vi "Main_Transmitter.vi"(8 "error in (no error)":errorcluster, 10 "Packet Parameters in":T3={"Length of sync sequence (50)"=50, "Number of message bits"=2048, "Number of guardbits"=30, "Sync PN sequence order (31)"=31, "Number of header bits"=16, "Packet Pad [samples]"=200}, 11 "QPSK System Parameters":T4={"Samples per Symbol"=8, "symbol map"=[], "Differential PSK"=enum."enable", "PSK type"=0, "M-PSK"=8} {"PSK type" items=["normal", "shifted", "offset"]; "symbol map" format="%.3f"}) -> (0 "error out":errorcluster)   [LabVIEW 2014]
uses:
  <vilib>/addons/Modulation/Digital/General/MT Generate Bits (Galois, PN Order).vi
  <vilib>/addons/Modulation/Digital/Support/Common/Validators/mod_Generate Bits Validate.vi
  <vilib>/addons/Modulation/Analog/support/mod_Set Error Source.vi
  <vilib>/addons/Modulation/Digital/General/subVIs/mod_Generate Bits PN Sequence.vi
  <vilib>/addons/Modulation/Digital/General/MT Format Eye Diagram (complex).vi
  <instrlib>/niUSRP/niUSRP Write Tx Data (CDB Cluster).vi
  <vilib>/addons/Modulation/niDMT.lvlib
panel:
  out "Time to modulate packet [ms]":dbl
  in  "Test Setup":T1={"Packets to send"=100, "Queue Length"=10, "PN sequence order (9)"=9}
  in  "I/Q (I)":enum16{"I", "Q"}(ring) caption="Eye Diagram I/Q"
  out "Eye Diagram":cluster{"t0":dbl, "dt":dbl, "Y":dbl[]}[](graph)
  in  "autoscale":bool
  out "Constellation Graph":T2(graph)
  out "Frame transfer time [ms]":dbl
  out "Frame length [samples]":i32
  out "Effective bit rate [bits/s]":dbl
  out "Real Frames Sent":i32
  out "Blank Frames Sent":i32
  out "Time to transfer packet [ms]":dbl
  in  "stop 2":bool caption="stop"
  in  "Bits per sample":i32=16
  in  "Audio record time/delay (ms)":i32=200
  in  "Audio sample rate (Fs)":i32=6000
  in  "filter parameters":T5={"Alpha"=0.5, "Filter Length"=6, "TX Filter"=enum."Root Raised Cos"} {"Alpha" format="%.2f"}
  in  "USRP IP address":refnum<k15>="192.168.10.1"
  in  "Tx Parameters":T6={"Tx IQ Sampling\nRate [s/sec]"=400000.0, "Tx Frequency [Hz]"=2450000000.0, "Tx Gain [dB]"=0.0, "Tx Antenna"="TX1"} {"Tx Gain [dB]" format="%#.6p"; "Tx Frequency [Hz]" format="%#.6p"; "Tx IQ Sampling\nRate [s/sec]" format="%#.6p"}
  out "Actual Tx Parameters":T6={"Tx IQ Sampling\nRate [s/sec]"=400000.0, "Tx Frequency [Hz]"=915000000.0, "Tx Gain [dB]"=0.0, "Tx Antenna"="TX1"} {"Tx Gain [dB]" format="%#.6p"; "Tx Frequency [Hz]" format="%#.6p"; "Tx IQ Sampling\nRate [s/sec]" format="%#.6p"}
  # "Calculated values"
  # "Measurements"
  # "Graph Setup"
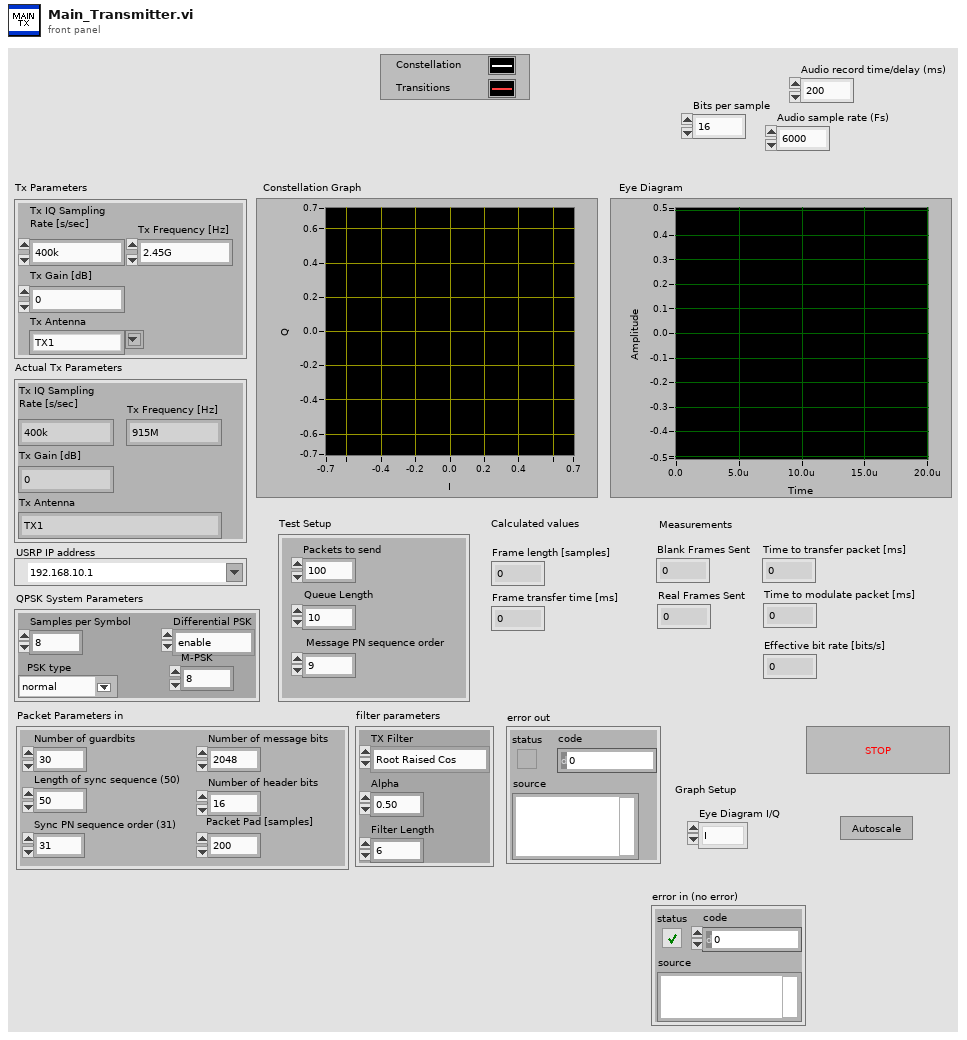
[diagram p1: front panel]
types:
  T1 = cluster{"Packets to send":i32, "Queue Length":i32, "PN sequence order (9)":i32}
  T2 = cluster{"Decimated Array":dbl[], "Decimated Array":dbl[]}[]
  T3 = cluster{"Length of sync sequence (50)":i32, "Number of message bits":i32, "Number of guardbits":i32, "Sync PN sequence order (31)":i32, "Number of header bits":i32, "Packet Pad [samples]":i32}
  T4 = cluster{"Samples per Symbol":i32, "symbol map":cdb[], "Differential PSK":enum16{"disable", "enable"}, "PSK type":u16, "M-PSK":i32}
  T5 = cluster{"Alpha":dbl, "Filter Length":i32, "TX Filter":enum16{"none", "Raised Cosine", "Root Raised Cos", "Gaussian"}}
  T6 = cluster{"Tx IQ Sampling\nRate [s/sec]":dbl, "Tx Frequency [Hz]":dbl, "Tx Gain [dB]":dbl, "Tx Antenna":string}
  T7 = cluster{"samples per symbol (16)":i32, "symbol map":cdb[], "differential PSK":enum16{"disable", "enable"}, "PSK type":u16}
  T8 = cluster{"s? t:f":cluster{"t0":dbl, "dt":dbl, "Y":cdb[]}, i32}
  T9 = typedef "niAMT.lvlib/Complex Data Waveform.ctl" = cluster{"t0":dbl, "dt":dbl, "Y":cdb[]}
  T10 = cluster{"constellation":dbl[], "oversampled data":dbl[]}[]
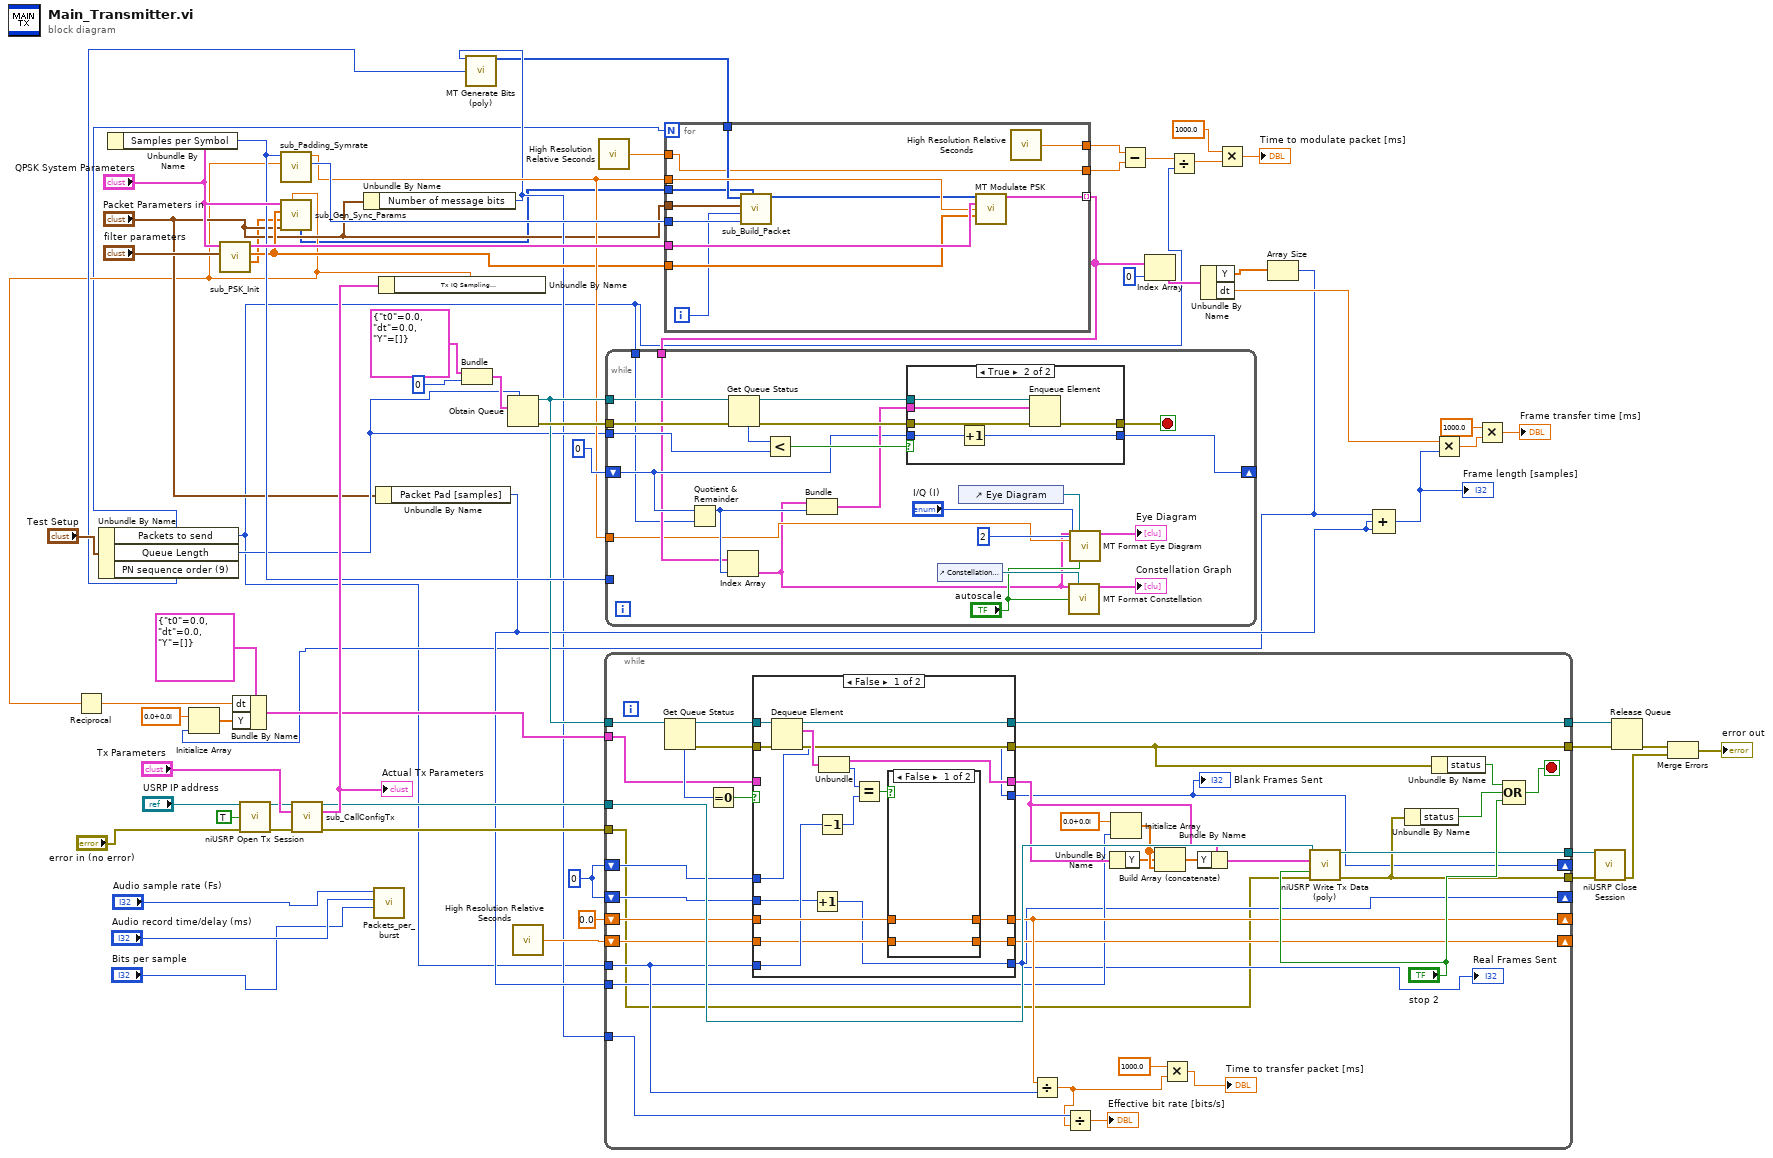
[diagram p0: block diagram]
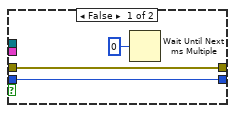
[diagram p2: hidden frame]
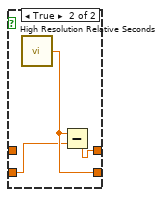
[diagram p3: hidden frame]
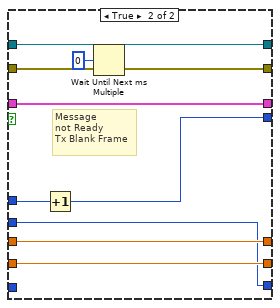
[diagram p4: hidden frame]
diagram:
  w31 = 0
  n1 = Unbundle By Name("Test Setup") -> ("Packets to send"=w6:i32, "Queue Length"=w18:i32, "PN sequence order (9)"=w17:i32)
  n2 = Unbundle By Name("QPSK System Parameters") -> ("Samples per Symbol"=w47:i32)
  n3 = call "sub_PSK_Init.vi"("filter parameters in"="filter parameters", "QPSK System Parameters in"="QPSK System Parameters") -> ("matched filter coefficients"=w11:dbl[], "pulse shaping filter coefficients"=w20:dbl[], "PSK system parameters"=w53:T7)  [unwired: 7 in]
  n4 = call <instrlib>:"niUSRP Open Tx Session.vi"("device names"="USRP IP address", "reset"=TRUE, "error in (no error)"="error in (no error)") -> ("session handle out"=w67:refnum<k15>, "error out"=w66:errorcluster)  [unwired: 11 in]
  n5 = call "sub_CallConfigTx.vi"("session handle"=w67, "Tx Parameters"="Tx Parameters", "error in"=w66) -> ("session handle out"=w61:refnum<k15>, "Actual Tx Parameters"=w62:T6, "error out"=w63:errorcluster)  [unwired: 10 in]
  "Actual Tx Parameters" <- w62
  n6 = Unbundle By Name("Packet Parameters in") -> ("Number of message bits"=w14:i32)
  n7 = call "Packets_per_burst.vi"("Bits per sample"="Bits per sample", "Audio record time/delay (ms)"="Audio record time/delay (ms)", "Audio sample rate (Fs)"="Audio sample rate (Fs)") -> ()  [unwired: 8 in, 1 out]
  n8 = Unbundle By Name("Packet Parameters in") -> ("Packet Pad [samples]"=w22:i32)
  n9 = Unbundle By Name(w62) -> ("Tx IQ Sampling\nRate [s/sec]"=w10:dbl)
  n10 = Reciprocal(x=w10) -> (1/x=w43:dbl)
  n11 = call "sub_Padding_Symrate.vi"("Tx IQ Sampling\nRate [s/sec]"=w10, "Samples per Symbol"=w47) -> ("Padding Bits"=w54:i32, "Symbol Rate"=w21:dbl)  [unwired: 8 in]
  n12 = call "sub_Gen_Sync_Params.vi"("IQ Sampling\nRate [s/sec]"=w10, "Packet Parameters in"="Packet Parameters in", "matched filter coefficients"=w11, "pulse shaping filter coefficients"=w20, "QPSK System Parameters in"="QPSK System Parameters") -> ("Sync Sequence Bitstream"=w1:i8[])  [unwired: 2 in, 4 out]
  n13 = Bundle("s? t:f"=cluster{"t0":dbl, "dt":dbl, "Y":cdb[]} {"t0"=0.0, "dt"=0.0, "Y"=[]}, 0) -> (w51:T8)  [unwired: 1 in]
  n14 = call-poly <vilib>:"MT Generate Bits (poly).vi"("total bits (128)"=w14, "PN sequence order (9)"=w17) -> ("output bit stream"=w13:i8[])  [unwired: 11 in, 2 out]
  n15 = Obtain Queue(max queue size (-1, unlimited)=w18, element data type=w51) -> (queue out=w46:refnum<queue>, error out=w49:errorcluster)  [unwired: 3 in, 1 out]
  n16 = call <vilib>:"High Resolution Relative Seconds.vi"() -> ("relative seconds"=w33:dbl)
  n17 = call <vilib>:"High Resolution Relative Seconds.vi"() -> ("relative seconds"=w9:dbl)
  n18 = for {
    N: w6 -> [_]
    tunnel: w54 -> [w80]
    tunnel: w53 -> [w79]
    tunnel: w21 -> [w78]
    tunnel: w20 -> [w77]
    tunnel: [w76] -> w30 mode=indexing
    tunnel: "Packet Parameters in" -> [w75]
    tunnel: w13 -> [w73]
    tunnel: w9 -> [w70]
    tunnel: [w71] -> w8
    tunnel: [w70] -> w7
    tunnel: w1 -> [w69]
    i -> [w72]
    n19 = call "sub_Build_Packet.vi"("Sync Sequence Bitstream"=w69, "Cyclic Padding Bits"=w80, "Packet number"=w72, "Packet Parameters in"=w75, "Input Message"=w73) -> ("Packet out"=w74:i8[])  [unwired: 6 in]
    n20 = call <vilib>:"MT Modulate PSK.vi"("input bit stream"=w74, "PSK system parameters"=w79, "symbol rate (Hz)"=w78, "pulse shaping filter coefficients"=w77) -> ("output complex waveform"=w76:T9)  [unwired: 9 in, 2 out]
    n21 = call <vilib>:"High Resolution Relative Seconds.vi"() -> ("relative seconds"=w71:dbl)
  }
  n22 = while {
    tunnel: w46 -> [w97]
    tunnel: w49 -> [w96]
    tunnel: w18 -> [w95]
    tunnel: w30 -> [w92]
    tunnel: w47 -> [_]
    tunnel: w6 -> [w91]
    shift-right: [w90] -> _
    shift-left: 0 -> [w94]
    tunnel: w21 -> [w83]
    stop <- w93 stop-if-true
    n23 = Quotient & Remainder(x=w94, y=w91) -> (x-y*floor(x/y)=w98:i32)  [unwired: 1 out]
    n24 = Index Array(array=w92, index=w98) -> (element=w81:T9)
    n25 = Get Queue Status(queue=w97, error in (no error)=w96) -> (queue out=w103:refnum<queue>, error out=w100:errorcluster, # elements in queue=w102:i32)  [unwired: 1 in, 5 out]
    n26 = Less?(x=w102, y=w95) -> (x < y?=w101:bool)
    n27 = Bundle("output complex waveform"=w81, w98) -> (w99:cluster{"output complex waveform":T9, i32})  [unwired: 1 in]
    n28 = case shown="True" w101 {
      tunnel: w100 -> [w104 w112]
      tunnel: w103 -> [_ w111]
      tunnel: [w104 w110] -> w93
      tunnel: w99 -> [_ w109]
      tunnel: w94 -> [w106 w108]
      tunnel: [w106 w107] -> w90
      frame False {
        n29 = Wait Until Next ms Multiple(millisecond multiple=u32 0) -> ()  [unwired: 1 out]
      }
      frame True {
        n30 = Increment(x=w108) -> (x+1=w107:i32)
        n31 = Enqueue Element(queue=w111, element=w109, error in (no error)=w112) -> (error out=w110:errorcluster)  [unwired: 1 in, 2 out]
      }
    }
    n32 = control-ref of="Constellation Graph"() -> (w86:refnum<vi>)
    n33 = control-ref of="Eye Diagram"() -> (w88:refnum<vi>)
    n34 = call <vilib>:"MT Format Constellation.vi"("waveform"=w81, "constellation reference"=w86, "autoscale"="autoscale") -> ("constellation graph"=→"Constellation Graph":T10)  [unwired: 2 in, 10 out]
    n35 = call-poly <vilib>:"MT Format Eye Diagram.vi"("waveform"=w81, "eye diagram reference"=w88, "symbol rate (Hz)"=w83, "eye length"=2, "I/Q (I)"="I/Q (I)", "autoscale"="autoscale") -> ("eye diagram"=→"Eye Diagram":cluster{"t0":dbl, "dt":dbl, "Y":dbl[]}[])  [unwired: 1 in, 8 out]
  }
  n36 = Subtract(x=w8, y=w7) -> (x-y=w5:dbl)
  n37 = Index Array(array=w30, index=0) -> (element=w28:T9)
  n38 = Divide(x=w5, y=w6) -> (x/y=w4:dbl)
  n39 = Unbundle By Name(w28) -> ("Y"=w27:cdb[], "dt"=w26:dbl)
  n40 = Multiply(x=1000.0, y=w4) -> (x*y=→"Time to modulate packet [ms]":dbl)
  n41 = Array Size(array=w27) -> (size(s)=w15:i32)
  n42 = Initialize Array(cdb 0.0+0.0i ("element"), w15) -> (w44:cdb[])
  n43 = Bundle By Name(cluster=cluster{"t0":dbl, "dt":dbl, "Y":cdb[]} {"t0"=0.0, "dt"=0.0, "Y"=[]} ("s? t:f"), "dt"=w43, "Y"=w44) -> (w41:cluster{"t0":dbl, "dt":dbl, "Y":cdb[]})
  n44 = while {
    tunnel: w63 -> [w113]
    tunnel: w61 -> [w140]
    tunnel: w46 -> [w142]
    tunnel: w41 -> [w141]
    tunnel: [w138] -> w37
    tunnel: [w137] -> w36
    tunnel: [w136] -> w35
    tunnel: [w135] -> w34
    shift-right: [w133] -> _
    shift-left: 0.0 -> [w134]
    tunnel: w6 -> [w132]
    shift-right: [w131] -> _
    shift-left: w33 -> [w130]
    shift-right: [w117] -> _
    shift-left: w31 -> [w129]
    shift-right: [w116] -> _
    shift-left: w31 -> [w128]
    tunnel: w14 -> [w127]
    tunnel: w22 -> [w121]
    stop <- w139 stop-if-true
    n45 = Get Queue Status(queue=w142) -> (queue out=w147:refnum<queue>, error out=w146:errorcluster, # elements in queue=w149:i32)  [unwired: 2 in, 5 out]
    n46 = Equal To 0?(x=w149) -> (x = 0?=w148:bool)
    n47 = case shown="False" w148 {
      tunnel: w141 -> [_ w180]
      tunnel: [w162 w180] -> w122
      tunnel: [w166 w178] -> w138
      tunnel: [w161 w179] -> w137
      tunnel: w147 -> [w165 w178]
      tunnel: w146 -> [w164 w179]
      tunnel: w134 -> [w158 w176]
      tunnel: [w157 w176] -> w133
      tunnel: w132 -> [w155 _]
      tunnel: [w154 w175] -> w131
      tunnel: w130 -> [w153 w175]
      tunnel: w129 -> [w152 w174]
      tunnel: [w152 w173] -> w117
      tunnel: w128 -> [w151 w172]
      tunnel: [w150 w172] -> w116
      frame False {
        n48 = Dequeue Element(queue=w165, error in (no error)=w164) -> (queue out=w166:refnum<queue>, element=w163:T8, error out=w161:errorcluster)  [unwired: 1 in, 1 out]
        n49 = Increment(x=w151) -> (x+1=w150:i32)
        n50 = Decrement(x=w155) -> (x-1=w156:i32)
        n51 = Unbundle(w163) -> ("s? t:f"=w162:cluster{"t0":dbl, "dt":dbl, "Y":cdb[]}, w159:i32)
        n52 = Equal?(x=w159, y=w156) -> (x = y?=w160:bool)
        n53 = case shown="False" w160 {
          tunnel: w158 -> [w167 _]
          tunnel: [w167 w171] -> w157
          tunnel: [w168 w170] -> w154
          tunnel: w153 -> [w168 w169]
          frame False {
          }
          frame True {
            n54 = call <vilib>:"High Resolution Relative Seconds.vi"() -> ("relative seconds"=w170:dbl)
            n55 = Subtract(x=w170, y=w169) -> (x-y=w171:dbl)
          }
        }
      }
      frame True {
        # "Message\nnot Ready\nTx Blank Frame"
        n56 = Increment(x=w174) -> (x+1=w173:i32)
        n57 = Wait Until Next ms Multiple(millisecond multiple=u32 0) -> ()  [unwired: 1 out]
      }
    }
    "Blank Frames Sent" <- w117
    "Real Frames Sent" <- w116
    n58 = Divide(x=w133, y=w132) -> (x/y=w119:dbl)
    n59 = Divide(x=w127, y=w119) -> (x/y=→"Effective bit rate [bits/s]":dbl)
    n60 = Unbundle By Name(w122) -> ("Y"=w123:cdb[])
    n61 = Initialize Array(cdb 0.0+0.0i ("element"), w121) -> (w124:cdb[])
    n62 = Build Array (concatenate)(w124, w123, w124) -> (w126:cdb[])
    n63 = Multiply(x=1000.0, y=w119) -> (x*y=→"Time to transfer packet [ms]":dbl)
    n64 = Bundle By Name(cluster=w122, "Y"=w126) -> (w118:cluster{"t0":dbl, "dt":dbl, "Y":cdb[]})
    n65 = call-poly <instrlib>:"niUSRP Write Tx Data (poly).vi"("session handle"=w140, "data"=w118, "end of data?"="stop 2", "error in (no error)"=w113) -> ("session handle out"=w136:refnum<k15>, "error out"=w135:errorcluster)  [unwired: 10 in]
    n66 = Unbundle By Name(w135) -> ("status"=w145:bool)
    n67 = Unbundle By Name(w137) -> ("status"=w143:bool)
    n68 = Compound Arithmetic op=OR(w143, w145, "stop 2") -> (w139:bool)
  }
  n69 = Compound Arithmetic op=ADD(w15, w22, w22) -> (w16:i32)
  "Frame length [samples]" <- w16
  n70 = Multiply(x=w26, y=w16) -> (x*y=w25:dbl)
  n71 = Multiply(x=1000.0, y=w25) -> (x*y=→"Frame transfer time [ms]":dbl)
  n72 = call <instrlib>:"niUSRP Close Session.vi"("session handle"=w35, "error in (no error)"=w34) -> ("error out"=w39:errorcluster)  [unwired: 13 in]
  n73 = Release Queue(queue=w37, error in (no error)=w36) -> (error out=w40:errorcluster)  [unwired: 3 out]
  n74 = Merge Errors(w40, w39) -> (→"error out":errorcluster)
